vi "maxLoop.vi"(11 "Loopkennung":u16[](array[numeric])) -> (3 "Numerisch":i32)   [LabVIEW 2020, in "PNS.lvlib"]
uses:
  PNS.lvlib
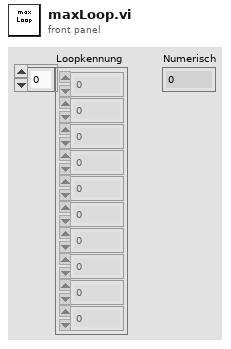
[diagram p1: front panel]
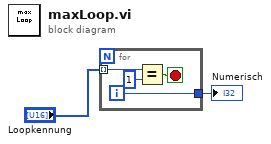
[diagram p0: block diagram]
diagram:
  n1 = for {
    tunnel: "Loopkennung" -> [w5] mode=indexing
    tunnel: [w3] -> w2
    i -> [w3]
    stop <- w6 stop-if-true
    n2 = Equal?(x=w5, y=u16 1) -> (x = y?=w6:bool)
  }
  "Numerisch" <- w2
